vi "PanelEngine.vi"() -> ()   [LabVIEW 2016, in "PCM PanelSplit.lvclass"]
uses:
  PCM PanelSplit.lvclass
  PanelSplitToolkit/PanelRootNode/PanelRootNode.lvclass
  C:/Users/CL/Desktop/ZcDAQprj0811/ZcDAQprj/Modules/DAQ-Display/PanelSplitToolkit/PanelDataNode/PanelDataNode.lvclass
  <vilib>/Utility/error.llb/DialogType.ctl
  PanelSplitToolkit/QueueManager.llb/Remove.vi
  PanelSplitToolkit/QueueManager.llb/Destroy.vi
  PanelSplitToolkit/QueueManager.llb/CreatQueue.vi
  PanelSplitToolkit/PanelDataNode/PanelDataNode.lvclass
panel:
  in  "LoaDefaultXML":bool=TRUE
  out "RootNode*":refnum<data-value>
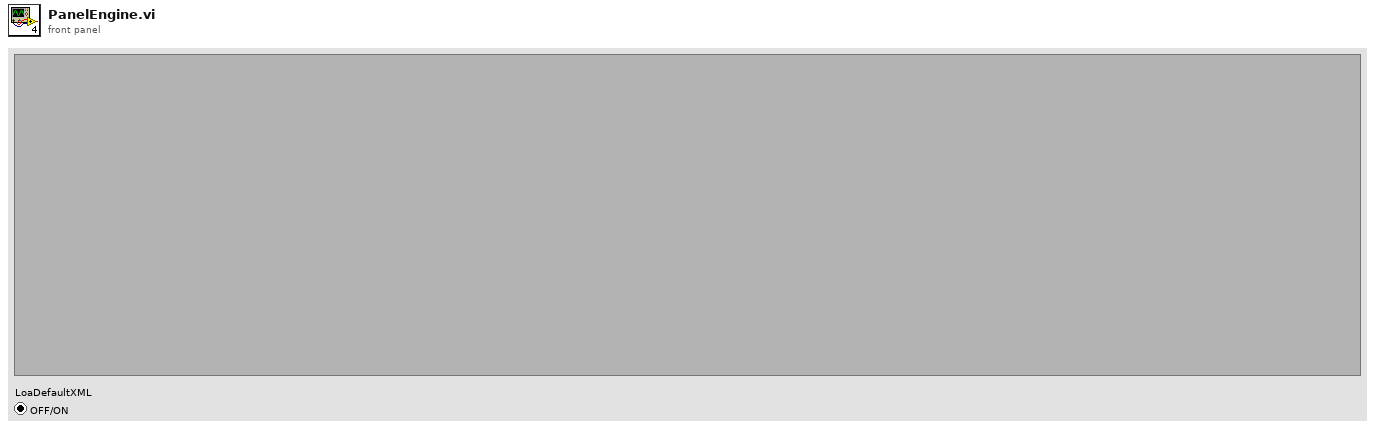
[diagram p1: front panel]
types:
  T1 = cluster{"error":errorcluster, "Event":string, "Data":variant, "Q_Local":string, "RootNode*":refnum<data-value>, "Caller":string}
  T2 = typedef "DialogType.ctl" = u16
  T3 = cluster{"TREE PNG":path, "User Guide":path, "DefaultSave":path, "BuildPath":path, "Image":path, "Modules":path, "Configuration":path, "License":path, "SplitFiles":path, "System.ini":path}
  T4 = typedef "Global para Config.ctl" = cluster{"连续存储设置":cluster{"Save Mode":i32, "Sel Save Mode":i32, "FolderPath":path, "Filename":string, "Explation":string, "AutoPoint":i32, "Template":path}, "Latest Prj":path, "Tdms Ref*":refnum<k34>, "默认波形图个数":u8, "列表列数":u8}
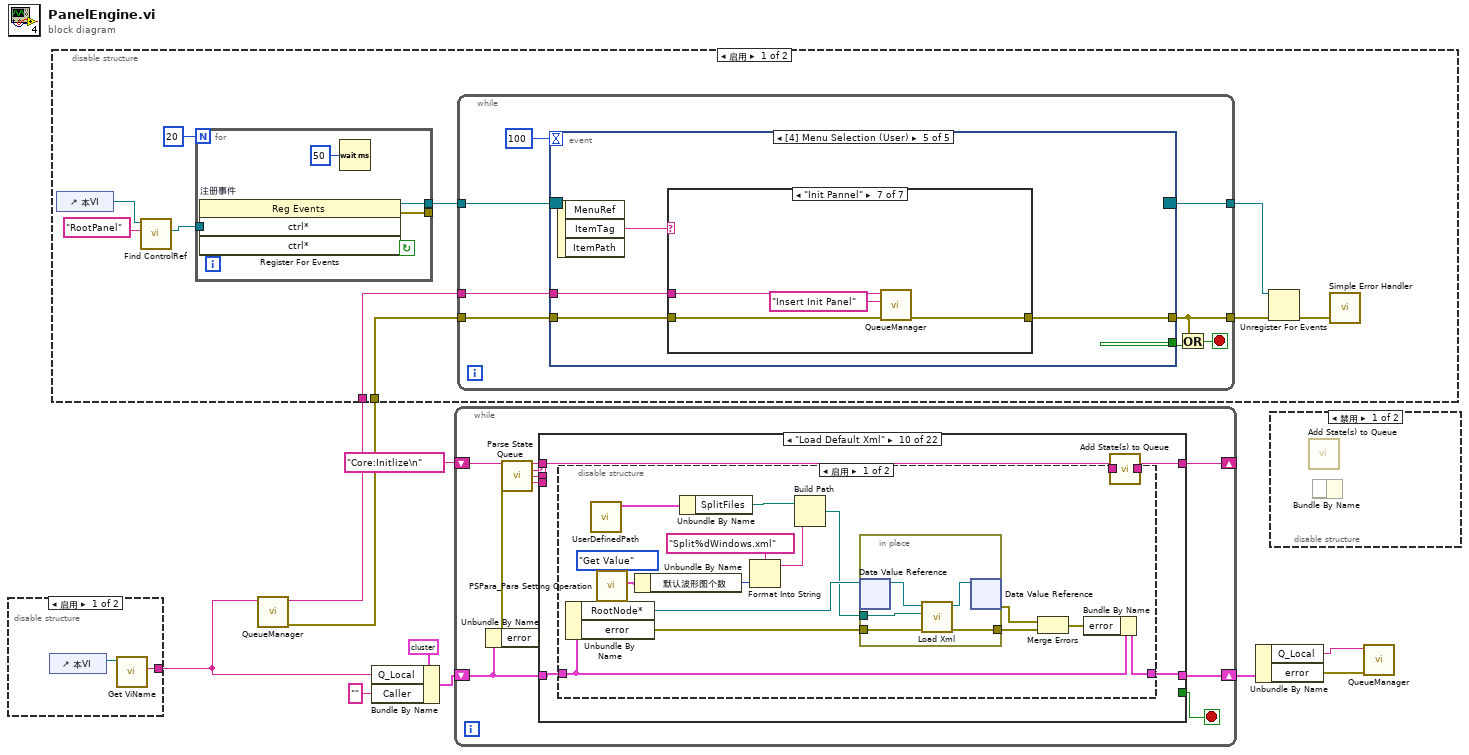
[diagram p0: block diagram]
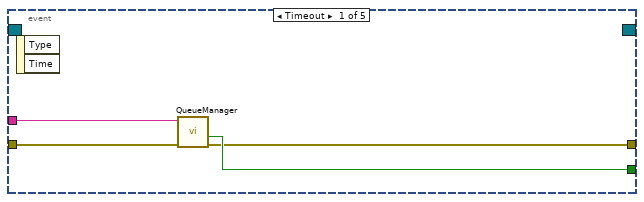
[diagram p2: hidden frame]
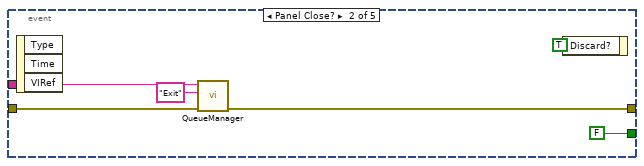
[diagram p3: hidden frame]
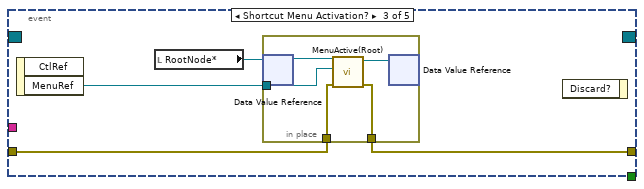
[diagram p4: hidden frame]
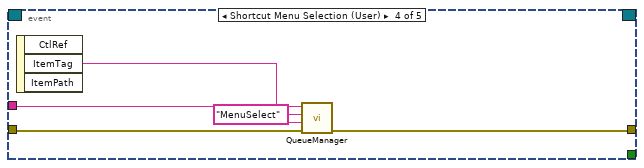
[diagram p5: hidden frame]
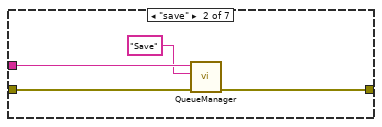
[diagram p7: hidden frame]
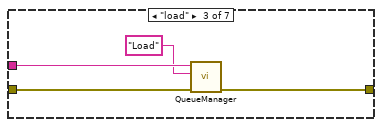
[diagram p8: hidden frame]
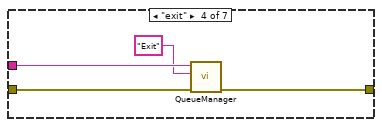
[diagram p9: hidden frame]
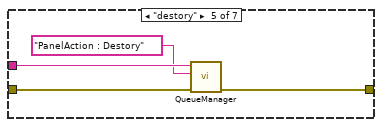
[diagram p10: hidden frame]
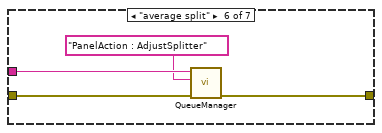
[diagram p11: hidden frame]
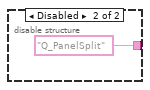
[diagram p13: hidden frame]
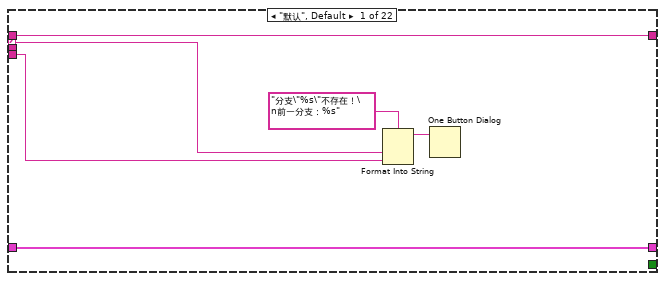
[diagram p15: hidden frame]
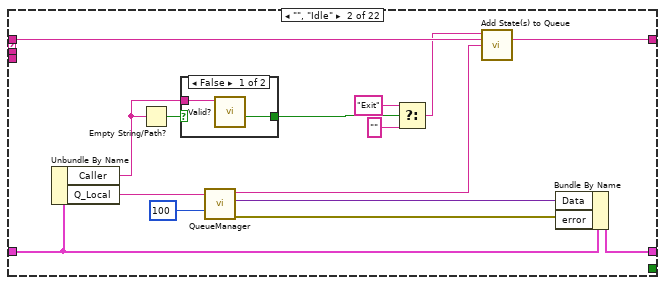
[diagram p16: hidden frame]
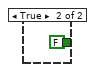
[diagram p17: hidden frame]
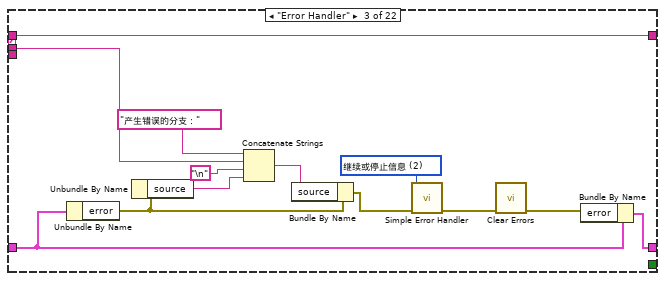
[diagram p18: hidden frame]
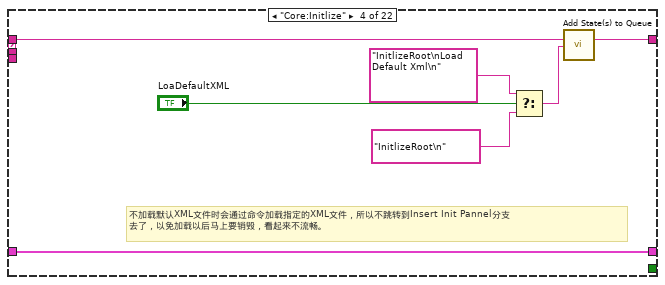
[diagram p19: hidden frame]
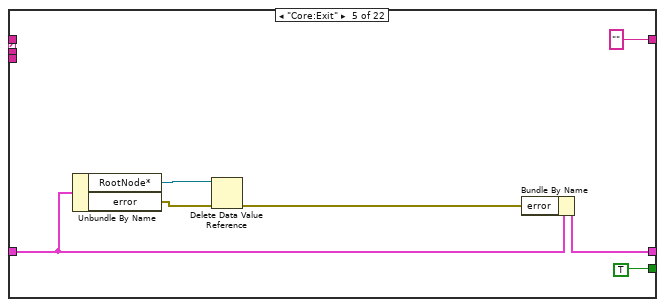
[diagram p20: hidden frame]
diagram:
  n1 = disable-structure shown="启用" {
    disable-tunnel: [w10 "Q_PanelSplit" ("QueueName")] -> w2
    frame Enabled {
      n2 = control-ref of="本VI"() -> (w11:refnum<vi>)
      n3 = call "Get ViName.vi"("VI*"=w11) -> ("VI Name"=w10:string)  [unwired: 8 in, 2 out]
    }
    frame Disabled {
    }
  }
  n4 = call-poly "QueueManager.vi"("QueueName"=w2) -> ("error out"=w9:errorcluster)  [unwired: 9 in, 1 out]
  n5 = disable-structure shown="启用" {
    disable-tunnel: w9 -> [w22 _]
    disable-tunnel: w2 -> [w21 _]
    frame Enabled {
      n6 = control-ref of="本VI"() -> (w20:refnum<vi>)
      n7 = call "Find ControlRef.vi"("control name"="RootPanel", "vi*"=w20) -> ("ctrl*"=w15:refnum<vi>)  [unwired: 7 in, 2 out]
      n8 = for {
        N: 20 -> [_]
        tunnel: [w24] -> _
        tunnel: [w26] -> w14
        tunnel: w15 -> [w25]
        stop <- w24 continue-if-true
        n9 = register-events "注册事件"(w25, w25) -> (reference out=w26:refnum<event-registration>, error out=w24:errorcluster)  [unwired: 2 in]
        n10 = Wait (ms)(milliseconds to wait=u32 50 ("等待时间（毫秒）")) -> ()  [unwired: 1 out]
      }
      n11 = while {
        tunnel: w22 -> [w33]
        tunnel: w21 -> [w34]
        tunnel: [w30] -> w18
        tunnel: w14 -> [w28]
        tunnel: [w27] -> w16
        stop <- w31 stop-if-true
        n12 = event shown="[4] Menu Selection (User)" {
          selector: w28 -> [_ _ _ _ _]
          dyn-events: [_ _ _ _ _] -> w27
          timeout: 100 -> [_ _ _ _ _]
          tunnel: [w36 FALSE _ _ _] -> w32
          tunnel: w34 -> [w38 w43 _ w58 w61]
          tunnel: w33 -> [w37 w42 w47 w57 w60]
          tunnel: [w35 w41 w48 w56 w59] -> w30
          event Timeout {
            n13 = event-data() -> ()  [unwired: 1 in, 2 out]
            n14 = call-poly "QueueManager.vi"("error in (no error)"=w37, "Queue Name(unamed)"=w38) -> ("error out"=w35:errorcluster, "Not Exist?"=w36:bool)  [unwired: 8 in]
          }
          event Panel Close? {
            n15 = event-data() -> ()  [unwired: 1 in, 3 out]
            n16 = call-poly "QueueManager.vi"("error in"=w42, "Event"="Exit", "QueueName"=w43) -> ("error out"=w41:errorcluster)  [unwired: 7 in, 1 out]
            n17 = event-data("Discard?"=TRUE ("放弃？")) -> ()  [unwired: 1 in, 1 out]
          }
          event Shortcut Menu Activation? {
            n18 = event-data() -> ("MenuRef"=w46:refnum<k9>)  [unwired: 1 in, 1 out]
            n19 = local read "RootNode*"() -> (w45:refnum<data-value>)
            n20 = in-place {
              in-place-border: w46 -> [w51]
              in-place-border: w47 -> [w50]
              in-place-border: [w49] -> w48
              n21 = in-place-dvr #1(w45) -> (w53:refnum<class "PanelRootNode.lvclass">)  [unwired: 1 out]
              n22 = call "MenuActive(Root).vi"("error in (no error)"=w50, "菜单引用"=w51, "PanelDataNode 输入"=w53) -> ("error out"=w49:errorcluster, "PanelDataNode 输出"=w52:refnum<class "PanelRootNode.lvclass">)  [unwired: 7 in]
              n23 = in-place-dvr #1(w52) -> ()  [unwired: 2 out]
            }
            n24 = event-data() -> ()  [unwired: 2 in, 1 out]
          }
          event Shortcut Menu Selection (User) {
            n25 = event-data() -> ("ItemTag"=w55:string)  [unwired: 1 in, 2 out]
            n26 = call-poly "QueueManager.vi"("error in"=w57, "Data"=w55, "Event"="MenuSelect", "QueueName"=w58) -> ("error out"=w56:errorcluster)  [unwired: 6 in, 1 out]
          }
          event Menu Selection (User) {
            n27 = event-data() -> ("ItemTag"=w62:string)  [unwired: 1 in, 2 out]
            n28 = case shown="\"Init Pannel\"" w62 {
              tunnel: w61 -> [_ w67 w71 w75 w79 w83 w85]
              tunnel: w60 -> [w63 w65 w69 w73 w77 w81 w87]
              tunnel: [w63 w64 w68 w72 w76 w80 w86] -> w59
              frame "假", Default {
              }
              frame "save" {
                n29 = call-poly "QueueManager.vi"("error in"=w65, "Event"="Save", "QueueName"=w67) -> ("error out"=w64:errorcluster)  [unwired: 7 in, 1 out]
              }
              frame "load" {
                n30 = call-poly "QueueManager.vi"("error in"=w69, "Event"="Load", "QueueName"=w71) -> ("error out"=w68:errorcluster)  [unwired: 7 in, 1 out]
              }
              frame "exit" {
                n31 = call-poly "QueueManager.vi"("error in"=w73, "Event"="Exit", "QueueName"=w75) -> ("error out"=w72:errorcluster)  [unwired: 7 in, 1 out]
              }
              frame "destory" {
                n32 = call-poly "QueueManager.vi"("error in"=w77, "Event"="PanelAction : Destory", "QueueName"=w79) -> ("error out"=w76:errorcluster)  [unwired: 7 in, 1 out]
              }
              frame "average split" {
                n33 = call-poly "QueueManager.vi"("error in"=w81, "Event"="PanelAction : AdjustSplitter", "QueueName"=w83) -> ("error out"=w80:errorcluster)  [unwired: 7 in, 1 out]
              }
              frame "Init Pannel" {
                n34 = call-poly "QueueManager.vi"("error in"=w87, "Event"="Insert Init Panel", "QueueName"=w85) -> ("error out"=w86:errorcluster)  [unwired: 7 in, 1 out]
              }
            }
          }
        }
        n35 = Or(x=w30, y=w32) -> (x .or. y?=w31:bool)
      }
      n36 = Unregister For Events(event registration refnum=w16, error in=w18) -> (error out=w17:errorcluster)
      n37 = call <vilib>:"Simple Error Handler.vi"("error in (no error)"=w17) -> ()  [unwired: 4 in, 5 out]
    }
    frame Disabled {
    }
  }
  n38 = Bundle By Name(cluster=T1 {"error"={"status"=FALSE, "code"=0, "source"=""}, "Event"="", "Data"=variant, "Q_Local"="", "RootNode*"=refnum, "Caller"=""} ("TmpData"), "Q_Local"=w2, "Caller"="") -> (w4:T1)
  n39 = while {
    shift-right: [w90] -> w6
    shift-left: w4 -> [w91]
    shift-right: [w89] -> _
    shift-left: "Core:Initlize\n" -> [w97]
    stop <- w93 stop-if-true
    n40 = Unbundle By Name(w91) -> ("error"=w92:errorcluster)
    n41 = call "Parse State Queue.vi"("State Queue"=w97, "Error In (no error)"=w92) -> ("Remaining States"=w96:string, "Current State"=w95:string, "Arguments"=w94:string, "PreState"=w88:string)  [unwired: 10 in]
    n42 = case shown="\"Load Default Xml\"" w95 {
      selector: w95 -> [w99 _ _ _ _ _ _ _ _ _ _ _ _ _ _ _ _ _ _ _ _ _]
      tunnel: w96 -> [w102 w114 w134 w140 _ w153 w154 w171 w183 w192 w224 w245 w263 w275 w286 w293 w307 w328 w338 w348 w354 w366]
      tunnel: w94 -> [_ _ w122 _ _ _ _ _ _ _ _ _ _ _ _ _ _ _ _ _ _ _]
      tunnel: [_ _ _ _ TRUE FALSE FALSE _ _ _ _ _ _ _ _ _ _ _ _ _ _ _] -> w93
      tunnel: w91 -> [w103 w111 w124 w141 w144 w150 w155 w164 w175 w190 w226 w243 w252 w279 w285 w292 w311 w326 w336 w346 w353 w364]
      tunnel: [w103 w117 w123 w141 w143 w150 w155 w166 w174 w189 w225 w242 w251 w278 w285 w291 w310 w325 w335 w345 w353 w363] -> w90
      tunnel: [w102 w113 w134 w139 "" ("Remaining States") w152 w154 w171 w183 w191 w224 w245 w263 w274 w286 w293 w306 w328 w338 w348 w354 w366] -> w89
      tunnel: w88 -> [w98 _ _ _ _ _ _ _ _ _ _ _ _ _ _ _ _ _ _ _ _ _]
      frame "默认", Default {
        n43 = Format Into String(format string="分支\"%s\"不存在！\n前一分支：%s" ("格式字符串"), w99, w98) -> (resulting string=w101:string)  [unwired: 2 in, 1 out]
        n44 = One Button Dialog(message=w101) -> ()  [unwired: 1 in, 1 out]
      }
      frame "", "Idle" {
        n45 = Unbundle By Name(w111) -> ("Caller"=w105:string, "Q_Local"=w110:string)
        n46 = Empty String/Path?(string/path=w105) -> (empty?=w109:bool)
        n47 = case shown="False" w109 {
          tunnel: [w120 FALSE ("Not Exist?")] -> w108
          tunnel: w105 -> [w119 _]
          frame False {
            n48 = call "Valid?.vi"("Queue Name(unamed)"=w119) -> ("Not Exist?"=w120:bool)  [unwired: 9 in, 1 out]
          }
          frame True {
          }
        }
        n49 = call-poly "QueueManager.vi"("Time out(-1)"=100, "Queue Name"=w110) -> ("error out"=w118:errorcluster, "Data"=w116:variant, "Event"=w115:string)  [unwired: 6 in, 1 out]
        n50 = Select(t="Exit" ("Event"), s=w108, f="") -> (s? t:f=w104:string)
        n51 = call "Add State(s) to Queue.vi"("State(s) in Front (\"\")"=w104, "State(s) in (\"\")"=w114, "State(s) at Back (\"\")"=w115) -> ("States Out"=w113:string)  [unwired: 12 in]
        n52 = Bundle By Name(cluster=w111, "Data"=w116, "error"=w118) -> (w117:T1)
      }
      frame "Error Handler" {
        w131 = T2 2 items=["无对话框", "确定信息", "继续或停止信息", "确定信息＋警告", "继续/停止+警告"] ("type of dialog (OK msg:1)")
        n53 = Unbundle By Name(w124) -> ("error"=w126:errorcluster)
        n54 = Unbundle By Name(w126) -> ("source"=w129:string)
        n55 = Concatenate Strings("产生错误的分支：" ("字符串"), w122, "\n", w129) -> (w127:string)
        n56 = Bundle By Name(cluster=w126, "source"=w127) -> (w125:errorcluster)
        n57 = call <vilib>:"Simple Error Handler.vi"("type of dialog (OK msg:1)"=w131, "error in (no error)"=w125) -> ("error out"=w132:errorcluster)  [unwired: 3 in, 4 out]
        n58 = call <vilib>:"Clear Errors.vi"("error in (no error)"=w132) -> ("error out"=w133:errorcluster)  [unwired: 5 in, 1 out]
        n59 = Bundle By Name(cluster=w124, "error"=w133) -> (w123:T1)
      }
      frame "Core:Initlize" {
        # "不加载默认XML文件时会通过命令加载指定的XML文件，所以不跳转到Insert Init Pannel分支\n去了，以免加载以后马上要销毁，看起来不流畅。"
        n60 = Select(t="InitlizeRoot\nLoad Default Xml\n" ("State(s) at Back (\"\")"), s="LoaDefaultXML", f="InitlizeRoot\n" ("State(s) at Back (\"\")")) -> (s? t:f=w136:string)
        n61 = call "Add State(s) to Queue.vi"("State(s) in (\"\")"=w140, "State(s) at Back (\"\")"=w136) -> ("States Out"=w139:string)  [unwired: 13 in]
      }
      frame "Core:Exit" {
        n62 = Unbundle By Name(w144) -> ("RootNode*"=w146:refnum<data-value>, "error"=w142:errorcluster)
        n63 = Delete Data Value Reference(data value reference=w146, error in=w142) -> (error out=w145:errorcluster)  [unwired: 1 out]
        n64 = Bundle By Name(cluster=w144, "error"=w145) -> (w143:T1)
      }
      frame "Exit" {
        n65 = call "Add State(s) to Queue.vi"("State(s) in (\"\")"=w153, "State(s) at Back (\"\")"="PanelAction : Destory\nCore:Exit" ("State(s) at Back (\"\")")) -> ("States Out"=w152:string)  [unwired: 13 in]
      }
      frame "------RootPanel-----------" {
      }
      frame "InitlizeRoot" {
        # ">> Notes: 初始化，注意将类替换掉<<"
        n66 = Unbundle By Name(w164) -> ("Q_Local"=w163:string, "error"=w158:errorcluster)
        n67 = control-ref of="本VI"() -> (w159:refnum<vi>)
        n68 = call "Find ControlRef.vi"("error in (no error)"=w158, "control name"="RootPanel", "vi*"=w159) -> ("error out"=w161:errorcluster, "ctrl*"=w160:refnum<vi>)  [unwired: 6 in, 1 out]
        n69 = To More Specific Class(target class=refnum<vi> refnum ("RootPanel"), reference=w160, error in=w161) -> (specific class reference=w169:refnum<vi>, error out=w168:errorcluster)
        n70 = call-dynamic "Initialize Root.vi"("RootQueueName"=w163, "error in (no error)"=w168, "CurrentVi*"=w159, "RootPanel*"=w169, "PanelRootNode 输入"=refnum<class "PCM PanelSplit.lvclass"> refnum ("PCM PanelSplit.lvclass")) -> ("error out"=w167:errorcluster, "SelfNode*"=w165:refnum<data-value>)  [unwired: 5 in]
        "RootNode*" <- w165
        n71 = Bundle By Name(cluster=w164, "RootNode*"=w165, "error"=w167) -> (w166:T1)
      }
      frame "Insert Init Panel" {
        n72 = Unbundle By Name(w175) -> ("RootNode*"=w176:refnum<data-value>, "error"=w177:errorcluster)
        n73 = vi-ref "PCM Panel With Menu UI.vi"() -> (w182:refnum<vi>)
        n74 = property class="VI"(reference=w182, error in=w177) -> (error out=w179:errorcluster, "Path"=w181:path)  [unwired: 1 out]
        n75 = call "Dynamic Load.vi"("error in"=w179, "Vi Path"=w181) -> ("错误输出"=w180:errorcluster, "vi reference"=w178:refnum<vi>)  [unwired: 8 in]
        n76 = in-place {
          in-place-border: w180 -> [w186]
          in-place-border: [w185] -> w172
          in-place-border: w178 -> [w184]
          n77 = in-place-dvr #2(w176) -> (w188:refnum<class "PanelRootNode.lvclass">)  [unwired: 1 out]
          n78 = call-dynamic "Insert Vi.vi"("error in (no error)"=w186, "VI*"=w184, "PanelDataNode 输入"=w188) -> ("error out"=w185:errorcluster, "PanelDataNode 输出"=w187:refnum<class "PanelRootNode.lvclass">)  [unwired: 7 in]
          n79 = in-place-dvr #2(w187) -> (w173:refnum<data-value>)  [unwired: 1 out]
        }
        n80 = Bundle By Name(cluster=w175, "RootNode*"=w173, "error"=w172) -> (w174:T1)
      }
      frame "Load Default Xml" {
        n81 = disable-structure shown="启用" {
          disable-tunnel: w192 -> [w209 _]
          disable-tunnel: [w208 "Insert Init Panel" ("States Out")] -> w191
          disable-tunnel: w190 -> [w203 w216]
          disable-tunnel: [w202 w216] -> w189
          frame Enabled {
            n82 = Unbundle By Name(w203) -> ("RootNode*"=w207:refnum<data-value>, "error"=w198:errorcluster)
            n83 = call "UserDefinedPath.vi"() -> ("UserDefinedPath"=w196:T3)  [unwired: 11 in]
            n84 = call "PSPara_Para Setting Operation.vi"("Operation"=enum16{"Set Value", "Get Value", "Initialize"}."Get Value") -> ("_Para"=w194:T4)  [unwired: 9 in, 1 out]
            n85 = Unbundle By Name(w194) -> ("默认波形图个数"=w193:u8)
            n86 = Unbundle By Name(w196) -> ("SplitFiles"=w201:path)
            n87 = Format Into String(format string="Split%dWindows.xml" ("格式字符串"), w193) -> (resulting string=w199:string)  [unwired: 2 in, 1 out]
            n88 = Build Path(base path=w201, name or relative path=w199) -> (appended path=w197:path)
            n89 = in-place {
              in-place-border: [w213] -> w205
              in-place-border: w197 -> [w211]
              in-place-border: w198 -> [w210]
              n90 = in-place-dvr #3(w207) -> (w212:refnum<class "PanelRootNode.lvclass">)  [unwired: 1 out]
              n91 = call-dynamic "Load Xml.vi"("error in"=w210, "selected path"=w211, "PanelRootNode 输入"=w212) -> ("error out"=w213:errorcluster, "PanelRootNode 输出"=w214:refnum<class "PanelRootNode.lvclass">)  [unwired: 7 in]
              n92 = in-place-dvr #3(w214) -> (w206:errorcluster)  [unwired: 1 out]
            }
            n93 = Merge Errors(w206, w205) -> (w204:errorcluster)
            n94 = Bundle By Name(cluster=w203, "error"=w204) -> (w202:T1)
            n95 = call "Add State(s) to Queue.vi"("State(s) in (\"\")"=w209) -> ("States Out"=w208:string)  [unwired: 14 in]
          }
          frame Disabled {
          }
        }
      }
      frame "Save" {
        # ">> Notes: 保存分割结果，可通过队列发送保存的路径，也可不发送路径，自动弹出文件选择对话框。<<"
        n96 = Unbundle By Name(w226) -> ("RootNode*"=w227:refnum<data-value>, "Data"=w222:variant, "error"=w217:errorcluster)
        n97 = Variant To Data(error in=w217, type=path "" ("路径"), Variant=w222) -> (data=w220:path, error out=w219:errorcluster)
        n98 = call <vilib>:"Clear Errors.vi"("error in (no error)"=w219) -> ("error out"=w218:errorcluster)  [unwired: 5 in, 1 out]
        n99 = in-place {
          in-place-border: [w230] -> w223
          in-place-border: w220 -> [w229]
          in-place-border: w218 -> [w228]
          n100 = in-place-dvr #4(w227) -> (w232:refnum<class "PanelRootNode.lvclass">)  [unwired: 1 out]
          n101 = call-dynamic "Save Xml.vi"("error in"=w228, "selected path"=w229, "PanelRootNode 输入"=w232) -> ("error out"=w230:errorcluster, "PanelRootNode 输出"=w231:refnum<class "PanelRootNode.lvclass">)  [unwired: 7 in]
          n102 = in-place-dvr #4(w231) -> ()  [unwired: 2 out]
        }
        n103 = Bundle By Name(cluster=w226, "error"=w223) -> (w225:T1)
      }
      frame "Load" {
        n104 = Unbundle By Name(w243) -> ("RootNode*"=w244:refnum<data-value>, "Data"=w239:variant, "error"=w236:errorcluster)
        n105 = Variant To Data(error in=w236, type=path "" ("路径"), Variant=w239) -> (data=w238:path, error out=w240:errorcluster)
        n106 = call <vilib>:"Clear Errors.vi"("error in (no error)"=w240) -> ("error out"=w237:errorcluster)  [unwired: 5 in, 1 out]
        n107 = in-place {
          in-place-border: [w249] -> w234
          in-place-border: w238 -> [w247]
          in-place-border: w237 -> [w246]
          n108 = in-place-dvr #5(w244) -> (w248:refnum<class "PanelRootNode.lvclass">)  [unwired: 1 out]
          n109 = call-dynamic "Load Xml.vi"("error in"=w246, "selected path"=w247, "PanelRootNode 输入"=w248) -> ("error out"=w249:errorcluster, "PanelRootNode 输出"=w250:refnum<class "PanelRootNode.lvclass">)  [unwired: 7 in]
          n110 = in-place-dvr #5(w250) -> (w235:errorcluster)  [unwired: 1 out]
        }
        n111 = Merge Errors(w235, w234) -> (w233:errorcluster)
        n112 = Bundle By Name(cluster=w243, "error"=w233) -> (w242:T1)
      }
      frame "LoadXmlString" {
        n113 = Unbundle By Name(w252) -> ("RootNode*"=w262:refnum<data-value>, "Q_Local"=w253:string, "Data"=w260:variant, "error"=w257:errorcluster)
        n114 = Variant To Data(error in=w257, type=w253, Variant=w260) -> (data=w259:string, error out=w261:errorcluster)
        n115 = call <vilib>:"Clear Errors.vi"("error in (no error)"=w261) -> ("error out"=w258:errorcluster)  [unwired: 5 in, 1 out]
        n116 = in-place {
          in-place-border: [w267] -> w255
          in-place-border: w259 -> [w264]
          in-place-border: w258 -> [w268]
          n117 = in-place-dvr #6(w262) -> (w266:refnum<class "PanelRootNode.lvclass">)  [unwired: 1 out]
          n118 = call-dynamic "LoadXmlString.vi"("error in"=w268, "XmlString"=w264, "PanelRootNode 输入"=w266) -> ("error out"=w267:errorcluster, "PanelRootNode 输出"=w265:refnum<class "PanelRootNode.lvclass">)  [unwired: 7 in]
          n119 = in-place-dvr #6(w265) -> (w256:errorcluster)  [unwired: 1 out]
        }
        n120 = Merge Errors(w256, w255) -> (w254:errorcluster)
        n121 = Bundle By Name(cluster=w252, "error"=w254) -> (w251:T1)
      }
      frame "MenuSelect" {
        n122 = Unbundle By Name(w279) -> ("RootNode*"=w273:refnum<data-value>, "Data"=w277:variant, "error"=w269:errorcluster)
        n123 = Variant To Data(error in=w269, type="", Variant=w277) -> (data=w272:string, error out=w271:errorcluster)
        n124 = in-place {
          in-place-border: w272 -> [w282]
          in-place-border: w271 -> [w281]
          in-place-border: [w280] -> w270
          n125 = in-place-dvr #7(w273) -> (w284:refnum<class "PanelRootNode.lvclass">)  [unwired: 1 out]
          n126 = call-dynamic "MenuSelect.vi"("error in"=w281, "Tag"=w282, "PanelRootNode 输入"=w284) -> ("error out"=w280:errorcluster, "PanelRootNode 输出"=w283:refnum<class "PanelRootNode.lvclass">)  [unwired: 7 in]
          n127 = in-place-dvr #7(w283) -> ()  [unwired: 2 out]
        }
        n128 = Bundle By Name(cluster=w279, "error"=w270) -> (w278:T1)
        n129 = call "Add State(s) to Queue.vi"("State(s) in (\"\")"=w275) -> ("States Out"=w274:string)  [unwired: 14 in]
      }
      frame "-------PanelAction----------" {
      }
      frame "PanelAction : Split" {
        n130 = Unbundle By Name(w292) -> ("RootNode*"=w290:refnum<data-value>, "Data"=w289:variant, "error"=w287:errorcluster)
        n131 = in-place {
          in-place-border: w289 -> [w297]
          in-place-border: [w296] -> w288
          in-place-border: w287 -> [w295]
          n132 = in-place-dvr #8(w290) -> (w299:refnum<class "PanelRootNode.lvclass">)  [unwired: 1 out]
          n133 = call-dynamic "Split.vi"("Average Splitter?"=TRUE, "error in"=w295, "Data"=w297, "PanelRootNode 输入"=w299) -> ("error out"=w296:errorcluster, "PanelRootNode 输出"=w298:refnum<class "PanelRootNode.lvclass">)  [unwired: 6 in]
          n134 = in-place-dvr #8(w298) -> ()  [unwired: 2 out]
        }
        n135 = Bundle By Name(cluster=w292, "error"=w288) -> (w291:T1)
      }
      frame "PanelAction : Delete" {
        # "保持子面板中至少插有一个VI。"
        n136 = Unbundle By Name(w311) -> ("RootNode*"=w312:refnum<data-value>, "Data"=w309:variant)
        n137 = in-place {
          in-place-border: w309 -> [w322]
          in-place-border: [w319] -> w308
          in-place-border: [w320] -> w302
          in-place-border: [w313] -> _
          n138 = in-place-dvr #9(w312) -> (w318:refnum<class "PanelRootNode.lvclass">)  [unwired: 1 out]
          n139 = call "Get LeafNodes[].vi"("PanelRootNode 输入"=w318) -> ("error out"=w316:errorcluster, "LeafNodes[]"=w315:refnum<data-value>[], "PanelRootNode 输出"=w317:refnum<class "PanelRootNode.lvclass">)  [unwired: 8 in]
          n140 = call-dynamic "Delete.vi"("Average Splitter?"=TRUE, "error in"=w316, "Data"=w322, "PanelRootNode 输入"=w317) -> ("error out"=w319:errorcluster, "PanelRootNode 输出"=w314:refnum<class "PanelRootNode.lvclass">)  [unwired: 6 in]
          n141 = Array Size(array=w315) -> (size(s)=w320:i32)
          n142 = call "Get LeafNodes[].vi"("PanelRootNode 输入"=w314) -> ("LeafNodes[]"=w313:refnum<data-value>[])  [unwired: 8 in, 2 out]
          n143 = in-place-dvr #9(w314) -> ()  [unwired: 2 out]
        }
        n144 = Equal?(x=w302, y=1) -> (x = y?=w300:bool)
        n145 = Select(t="Insert Init Panel" ("State(s) at Back (\"\")"), s=w300, f="") -> (s? t:f=w304:string)
        n146 = Bundle By Name(cluster=w311, "error"=w308) -> (w310:T1)
        n147 = call "Add State(s) to Queue.vi"("State(s) in (\"\")"=w307, "State(s) at Back (\"\")"=w304) -> ("States Out"=w306:string)  [unwired: 13 in]
      }
      frame "PanelAction : Insert" {
        n148 = Unbundle By Name(w326) -> ("RootNode*"=w327:refnum<data-value>, "Data"=w323:variant)
        n149 = in-place {
          in-place-border: [w329] -> w324
          in-place-border: w323 -> [w330]
          n150 = in-place-dvr #10(w327) -> (w332:refnum<class "PanelRootNode.lvclass">)  [unwired: 1 out]
          n151 = call-dynamic "Insert.vi"("Data"=w330, "PanelRootNode 输入"=w332) -> ("error out"=w329:errorcluster, "PanelRootNode 输出"=w331:refnum<class "PanelRootNode.lvclass">)  [unwired: 8 in]
          n152 = in-place-dvr #10(w331) -> ()  [unwired: 2 out]
        }
        n153 = Bundle By Name(cluster=w326, "error"=w324) -> (w325:T1)
      }
      frame "PanelAction : Destory" {
        # ">> Notes: 销毁分割结果，回到最初状态<<"
        n154 = Unbundle By Name(w336) -> ("RootNode*"=w337:refnum<data-value>, "error"=w333:errorcluster)
        n155 = in-place {
          in-place-border: [w340] -> w334
          in-place-border: w333 -> [w339]
          n156 = in-place-dvr #11(w337) -> (w342:refnum<class "PanelRootNode.lvclass">)  [unwired: 1 out]
          n157 = call-dynamic "Destory.vi"("error in (no error)"=w339, "PanelRootNode 输入"=w342) -> ("error out"=w340:errorcluster, "PanelRootNode 输出"=w341:refnum<class "PanelRootNode.lvclass">)  [unwired: 8 in]
          n158 = in-place-dvr #11(w341) -> ()  [unwired: 2 out]
        }
        n159 = Bundle By Name(cluster=w336, "error"=w334) -> (w335:T1)
      }
      frame "PanelAction : AdjustSplitter" {
        # ">> Notes: 均分面板<<"
        n160 = Unbundle By Name(w346) -> ("RootNode*"=w347:refnum<data-value>, "error"=w343:errorcluster)
        n161 = in-place {
          in-place-border: [w350] -> w344
          in-place-border: w343 -> [w349]
          n162 = in-place-dvr #12(w347) -> (w352:refnum<class "PanelRootNode.lvclass">)  [unwired: 1 out]
          n163 = call "Adjust Splitter.vi"("error in (no error)"=w349, "PanelRootNode 输入"=w352) -> ("error out"=w350:errorcluster, "PanelRootNode 输出"=w351:refnum<class "PanelRootNode.lvclass">)  [unwired: 8 in]
          n164 = in-place-dvr #12(w351) -> ()  [unwired: 2 out]
        }
        n165 = Bundle By Name(cluster=w346, "error"=w344) -> (w345:T1)
      }
      frame "------Communication---------" {
      }
      frame "SendToAllPanels" {
        # ">> Notes: 发送至所有面板中插入的VI线程，要求插入的VI使用的队列名是VI名称；<<"
        n166 = Unbundle By Name(w364) -> ("RootNode*"=w365:refnum<data-value>, "Data"=w361:variant, "error"=w355:errorcluster)
        n167 = Variant To Data(error in=w355, type=cluster{"Event":string, "Data":variant} {"Event"="", "Data"=variant}, Variant=w361) -> (data=w359:cluster{"Event":string, "Data":variant}, error out=w356:errorcluster)
        n168 = Unbundle By Name(w359) -> ("Event"=w358:string, "Data"=w357:variant)
        n169 = in-place {
          in-place-border: [w371] -> w362
          in-place-border: w358 -> [w370]
          in-place-border: w357 -> [w369]
          in-place-border: w356 -> [w368]
          n170 = in-place-dvr #13(w365) -> (w373:refnum<class "PanelRootNode.lvclass">)  [unwired: 1 out]
          n171 = call "SendToPanels.vi"("PanelNumber(-1)"=-1, "error in"=w368, "Data"=w369, "Event"=w370, "PanelRootNode in"=w373) -> ("error out"=w371:errorcluster, "PanelRootNode out"=w372:refnum<class "PanelRootNode.lvclass">)  [unwired: 5 in]
          n172 = in-place-dvr #13(w372) -> ()  [unwired: 2 out]
        }
        n173 = Bundle By Name(cluster=w364, "error"=w362) -> (w363:T1)
      }
    }
  }
  n174 = Unbundle By Name(w6) -> ("Q_Local"=w3:string, "error"=w7:errorcluster)
  n175 = disable-structure shown="禁用" {
    frame Disabled {
      n176 = call "Add State(s) to Queue.vi"() -> ()  [unwired: 15 in, 1 out]
      n177 = Bundle By Name() -> ()  [unwired: 2 in, 1 out]
    }
    frame Enabled {
    }
  }
  n178 = call-poly "QueueManager.vi"("error in (no error)"=w7, "QueeuName"=w3) -> ()  [unwired: 9 in, 1 out]
